vi "Keyence.Cmd.ErrorStatus.vi"(8 "error in (no error)":errorcluster, 9 "Timeout [ms] (1000)":i32=1000, 11 "connection ID":refnum<k5>) -> (0 "error out":errorcluster, 1 "error found":bool, 2 "Errors":T1[](array[typedef]), 3 "connection ID out":refnum<k5>)   [LabVIEW 2016]
uses:
  Keyence.ErrStat.ctl
panel:
  in  "error":T1
  out "response":string
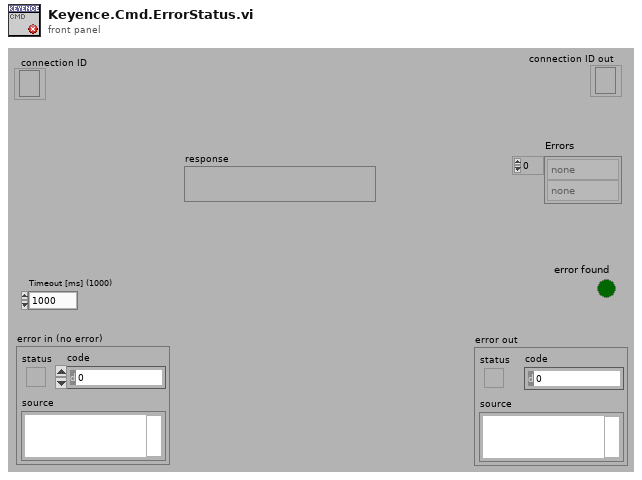
[diagram p1: front panel]
types:
  T1 = typedef "Keyence.ErrStat.ctl" = enum16{"none", "system", "update", "cfg", "ip", "over", "plc", "profinet", "lua", "undefined"}
  T2 = enum16{"Standard", "Buffered", "CRLF", "Immediate"}
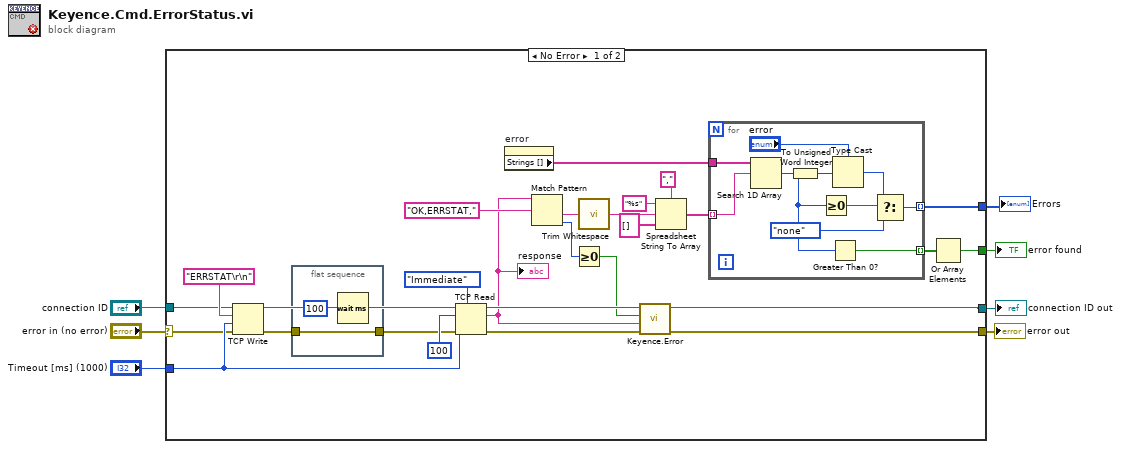
[diagram p0: block diagram]
diagram:
  n1 = case shown="No Error" "error in (no error)" {
    selector: "error in (no error)" -> [w11 w47]
    tunnel: [w25 w47] -> w7
    tunnel: "Timeout [ms] (1000)" -> [w33 _]
    tunnel: [w15 _] -> w4
    tunnel: [w13 _] -> w3
    tunnel: "connection ID" -> [w12 w46]
    tunnel: [w10 w46] -> w1
    frame No Error {
      n2 = TCP Write(connection ID=w12, data in="ERRSTAT\r\n" ("concatenated string"), error in (no error)=w11, 9:w33) -> (connection ID out=w32:refnum<k5>, error out=w29:errorcluster)  [unwired: 1 out]
      n3 = flat-sequence {
        tunnel: w29 -> [w45]
        tunnel: [w45] -> w28
        frame #0 {
          n4 = Wait (ms)(milliseconds to wait=u32 100) -> ()  [unwired: 1 out]
        }
      }
      n5 = TCP Read(connection ID=w32, bytes to read=100, error in (no error)=w28, 7:T2."Immediate" ("mode (standard)"), 9:w33) -> (connection ID out=w10:refnum<k5>, data out=w8:string, error out=w26:errorcluster)
      "response" <- w8
      n6 = property on="error" class="Enum (strict)"() -> ("Strings []"=w16:string[])  [unwired: 2 in, 2 out]
      n7 = Match Pattern(string=w8, regular expression="OK,ERRSTAT,") -> (after substring=w22:string, offset past match=w23:i32)  [unwired: 1 in, 2 out]
      n8 = Greater Or Equal To 0?(x=w23) -> (x >= 0?=w9:bool)
      n9 = call <vilib>:"Trim Whitespace.vi"("string"=w22) -> ("trimmed string"=w19:string)  [unwired: 1 in]
      n10 = call "Keyence.Error.vi"("error in (no error)"=w26, "Response"=w8, "Cmd ok"=w9) -> ("error out"=w25:errorcluster)  [unwired: 8 in]
      n11 = Spreadsheet String To Array(delimiter (Tab)=",", format string="%s", spreadsheet string=w19, array type (2D Dbl)=string[] []) -> (array=w17:string[])
      n12 = for {
        tunnel: w17 -> [w42] mode=indexing
        tunnel: w16 -> [w43]
        tunnel: [w36] -> w15 mode=indexing
        tunnel: [w34] -> w14 mode=indexing
        n13 = Search 1D Array(1D array=w43, element=w42) -> (index of element=w35:i32)  [unwired: 1 in]
        n14 = To Unsigned Word Integer(number=w35) -> (unsigned 16bit integer=w41:u16)
        n15 = Greater Or Equal To 0?(x=w35) -> (x >= 0?=w39:bool)
        n16 = Greater Than 0?(x=w35) -> (x > 0?=w34:bool)
        n17 = Type Cast(type="error", x=w41) -> (*(type *) &x=w38:T1)
        n18 = Select(t=w38, s=w39, f=Keyence.ErrStat."none" ("error")) -> (s? t:f=w36:T1)
      }
      n19 = Or Array Elements(Boolean array=w14) -> (logical OR=w13:bool)
    }
    frame Error {
    }
  }
  "error out" <- w7
  "Errors" <- w4
  "error found" <- w3
  "connection ID out" <- w1
